vi "DAS_Hub.vi"() -> ()   [LabVIEW 2012]
uses:
  <vilib>/Platform/TimedLoop/XDataNode/timing_clust.ctl
  <vilib>/Platform/TimedLoop/XDataNode/nitl_modes.ctl
  <vilib>/Platform/TimedLoop/XDataNode/wakeup.ctl
  <vilib>/platform/TimedLoop/XDataNode/XDataNode.xnode
  <vilib>/regexp/Match Regular Expression.xnode
  <vilib>/Platform/TimedLoop/XDataNode/XDNodeRunTimeDep.lvlib
panel:
  in  "Pixel Size (uM)":dbl
  in  "Magnification":dbl
  in  "Time Between Shots":i64=200
  out "Most Recent Image":dbl[][](graph)
  in  "DAS MODE":u16(ring)=1 items=["Bulb Trigger Mode"=1, "Free Run Mode"=2]
  out "DER Host":bool
  out "DB Server":bool
  out "ProEM Host":bool
  out "ProEM Slave":bool
  out "CoolSnap Slave":bool
  out "PixelFly Slave":bool
  in  "Send To DER?":enum32{"Send to DER", "Don't Send to DER"}(radio)
  in  "Save as .AIA?":enum32{"Save to File", "Don't Save to File"}(radio)
  out "Top of Chamber Monitor":dynamicdata(graph)
  out "Atoms":i32[][](graph)
  in  "stop":bool
  out "Dark Field":i32[][](graph)
  out "No Atoms":i32[][](graph)
  # "(COMING SOON)"
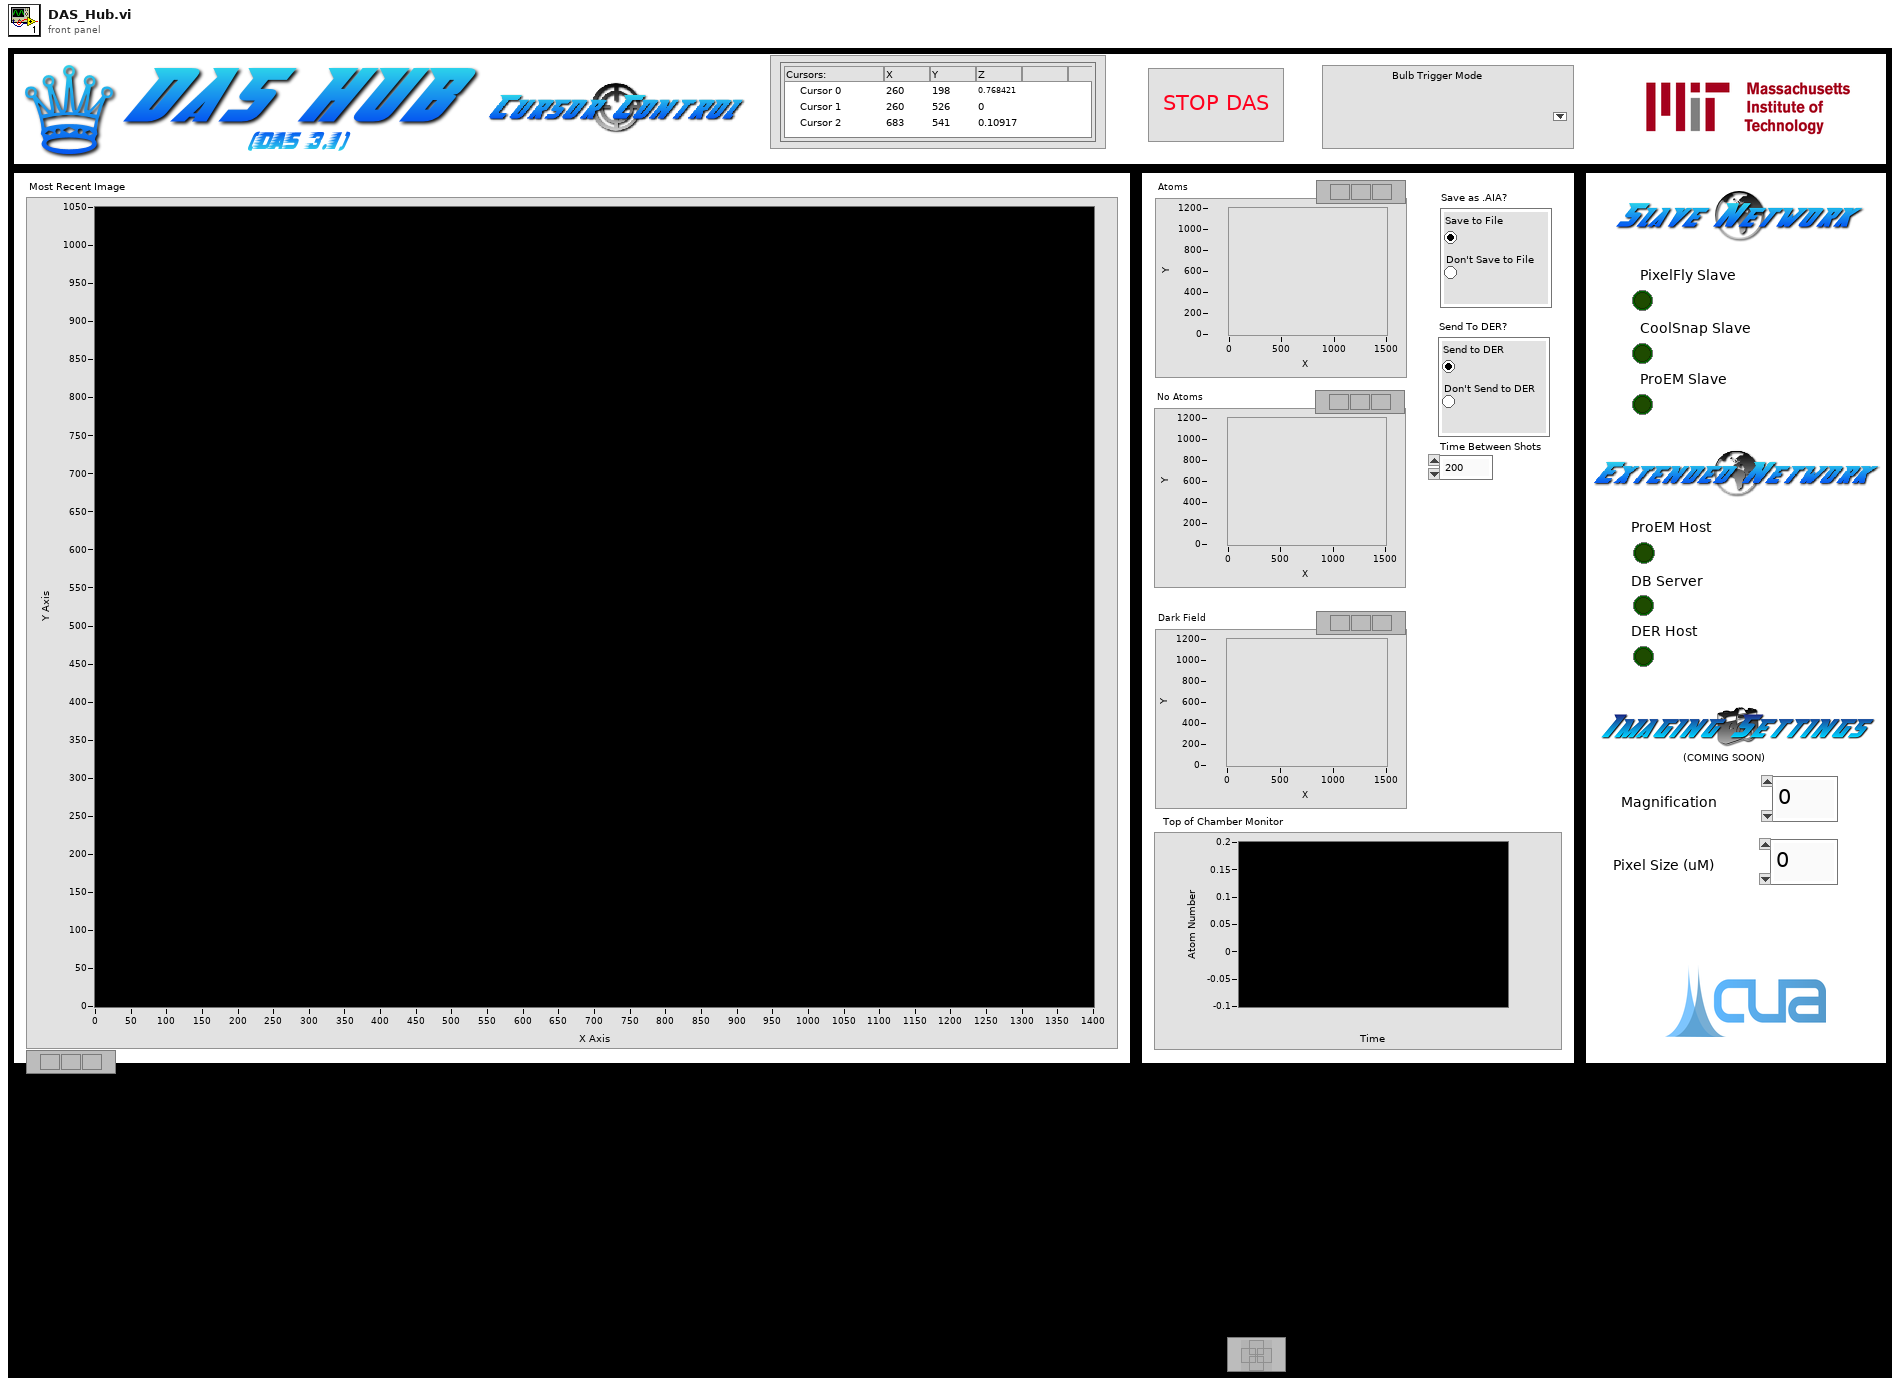
[diagram p1: front panel]
types:
  T1 = typedef "XDNodeRunTimeDep.lvlib/timing_clust.ctl" = cluster{"Expected End [f-1]":u64, "Actual End [f-1]":u64, "Finished Late? [f-1]":bool, "Expected End [i-1]":u64, "Actual End [i-1]":u64, "Finished Late? [i-1]":bool, "Expected Start [i]":u64, "Actual Start [i]":u64, "Expected Start [f]":u64, "Actual Start [f]":u64, "Source Name":string, "Structure Name":string, "Period":i64, "Deadline":i64, "Offset":i64, "Start":i64, "Priority":i32, "Timeout":i32, "Mode":T2, "Wakeup Reason":T3, "Error":errorcluster, "Source Type":string, "Secondary Source Type":string, "Global End Time":u64, "Global Start Time":u64, "Frame Duration":u64, "Iteration Duration":u64, "Assigned CPU":i32, "I/O Scan Engine Mode":u32}
  T2 = typedef "XDNodeRunTimeDep.lvlib/nitl_modes.ctl" = enum32{"No Change", "Process missed periods, maintain original phase", "Discard missed periods, maintain original phase", "Process missed periods, ignore original phase", "Discard missed periods, ignore original phase"}
  T3 = typedef "XDNodeRunTimeDep.lvlib/wakeup.ctl" = enum32{"Normal", "Aborted", "Asynchronous wakeup", "Timing source error", "Timed loop error", "Timeout"}
  T4 = typedef "LVDateTimeRec.ctl" = cluster{"fractional second":dbl, "second":i32, "minute":i32, "hour":i32, "day of month":i32, "month":i32, "year":i32, "day of week":i32, "day of year":i32, "DST":i32}
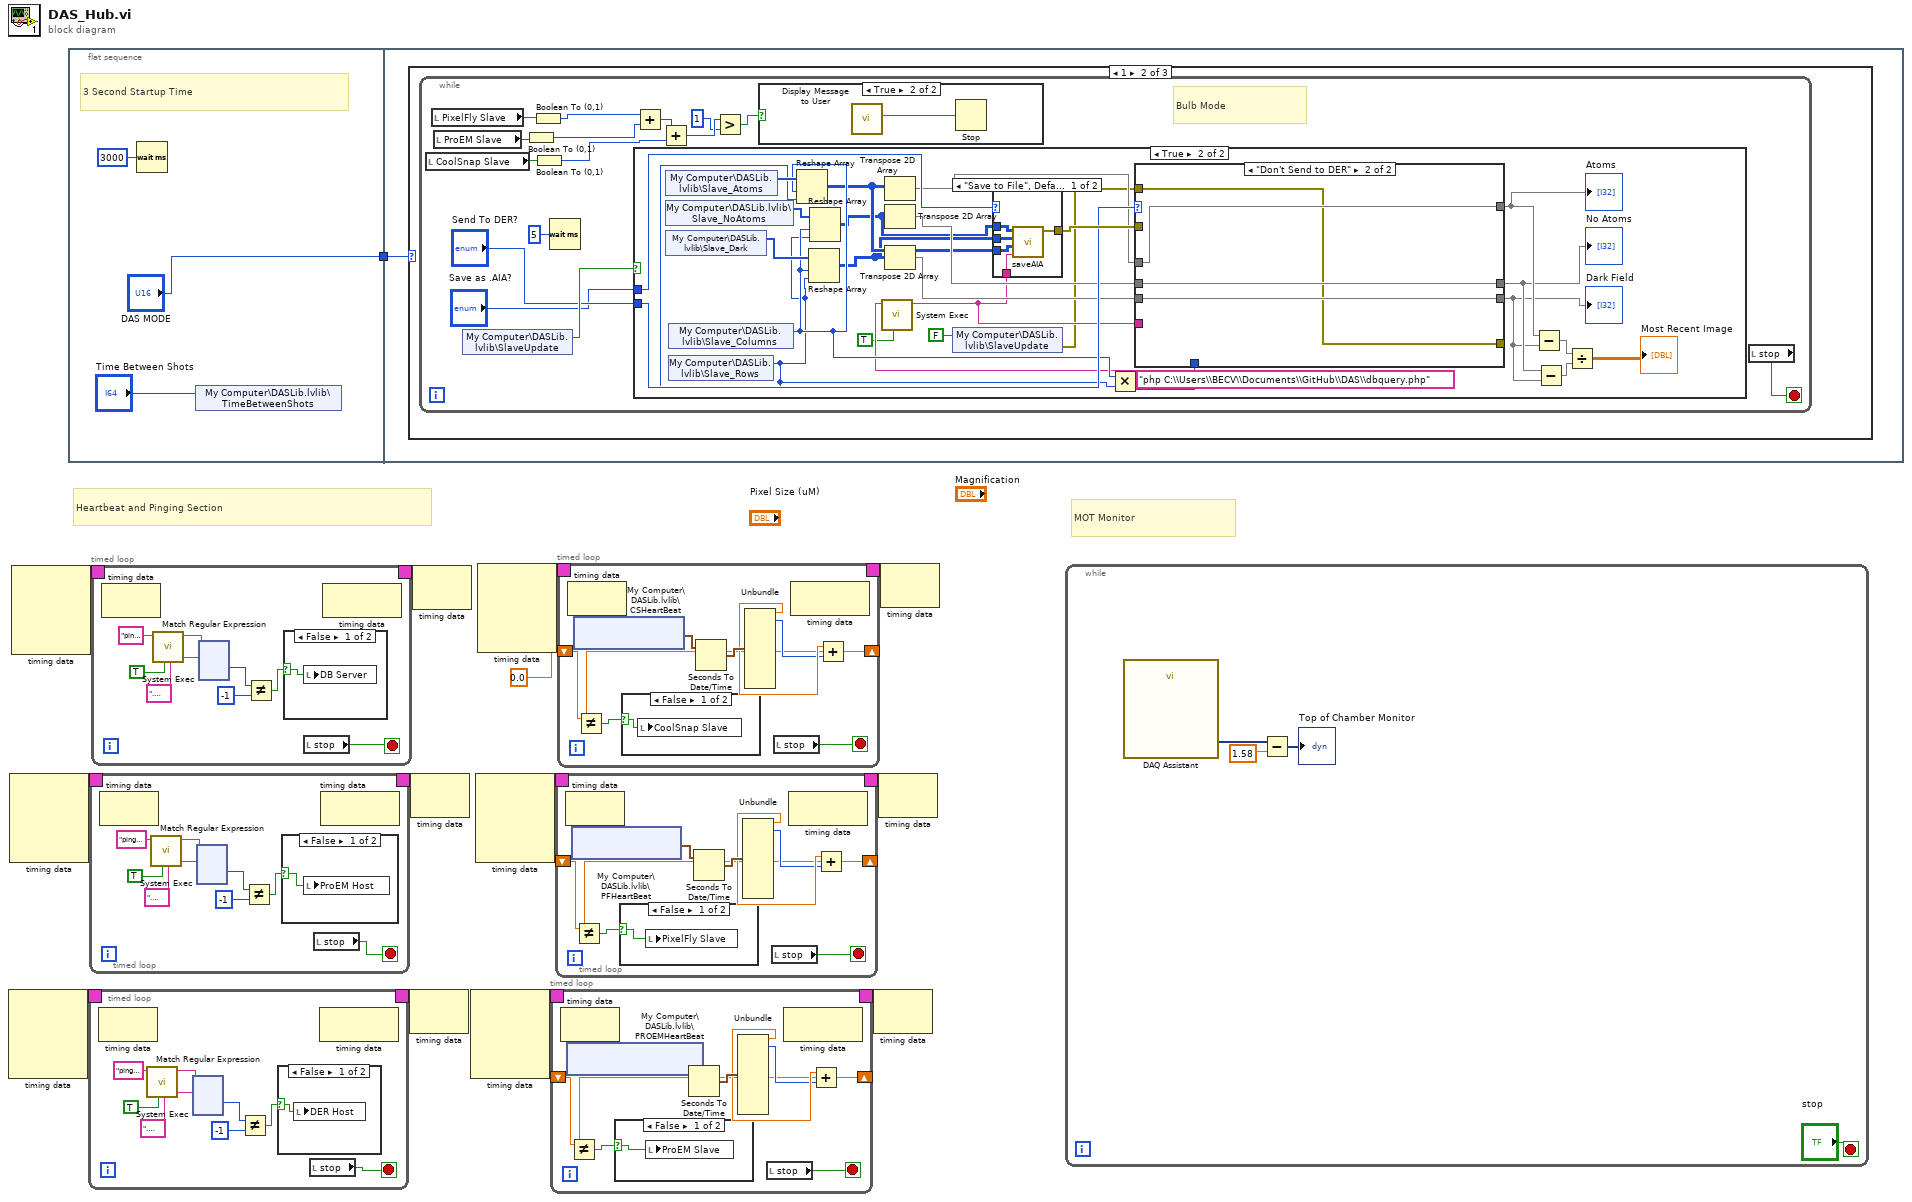
[diagram p0: block diagram]
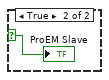
[diagram p2: hidden frame]
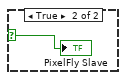
[diagram p3: hidden frame]
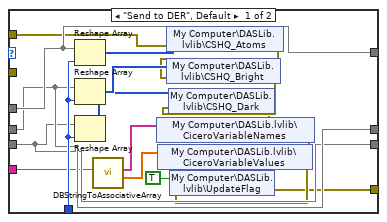
[diagram p7: hidden frame]
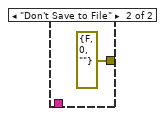
[diagram p8: hidden frame]
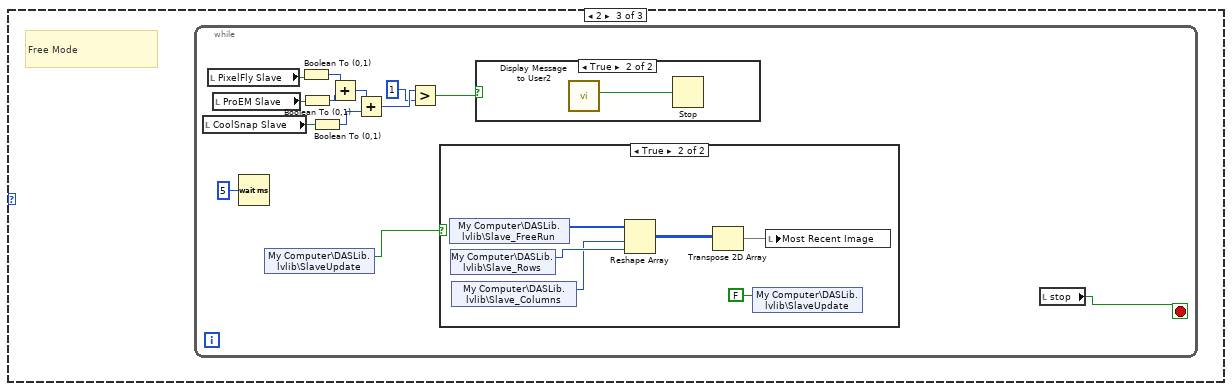
[diagram p9: hidden frame]
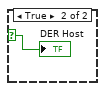
[diagram p12: hidden frame]
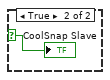
[diagram p13: hidden frame]
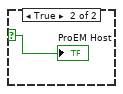
[diagram p14: hidden frame]
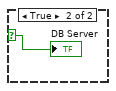
[diagram p15: hidden frame]
diagram:
  # "MOT Monitor"
  # "Heartbeat and Pinging Section"
  n1 = node-c288() -> (w8:T1)  [unwired: 4 in]
  n2 = node-c288() -> (w12:T1)  [unwired: 4 in]
  n3 = node-c288() -> (w14:T1)  [unwired: 4 in]
  n4 = flat-sequence {
    tunnel: ["DAS MODE"] -> w1
    tunnel: w1 -> [w18]
    frame #0 {
      # "3 Second Startup Time"
      n5 = Wait (ms)(milliseconds to wait=u32 3000) -> ()  [unwired: 1 out]
      n6 = shared-variable "My Computer\\DASLib.lvlib\\TimeBetweenShots"("Time Between Shots") -> ()  [unwired: 1 in, 1 out]
    }
    frame #1 {
      n7 = case shown="1" w18 {
        frame 0, Default {
          # "No-Camera Mode"
        }
        frame 1 {
          n8 = while {
            stop <- w29 stop-if-true
            # "Bulb Mode"
            n9 = local read "CoolSnap Slave"() -> (w26:bool)
            n10 = local read "PixelFly Slave"() -> (w28:bool)
            n11 = local read "ProEM Slave"() -> (w27:bool)
            n12 = shared-variable "My Computer\\DASLib.lvlib\\SlaveUpdate"() -> (w33:bool)  [unwired: 1 in, 1 out]
            n13 = Boolean To (0,1)(Boolean=w27) -> (0, 1=w24:i16)
            n14 = Boolean To (0,1)(Boolean=w28) -> (0, 1=w25:i16)
            n15 = Boolean To (0,1)(Boolean=w26) -> (0, 1=w23:i16)
            n16 = Wait (ms)(milliseconds to wait=u32 5) -> ()  [unwired: 1 out]
            n17 = case shown="True" w33 {
              tunnel: "Save as .AIA?" -> [_ w57]
              tunnel: "Send To DER?" -> [_ w55]
              frame False {
              }
              frame True {
                n18 = shared-variable "My Computer\\DASLib.lvlib\\Slave_Atoms"() -> (w60:i32[])  [unwired: 1 in, 1 out]
                n19 = shared-variable "My Computer\\DASLib.lvlib\\Slave_NoAtoms"() -> (w59:i32[])  [unwired: 1 in, 1 out]
                n20 = shared-variable "My Computer\\DASLib.lvlib\\Slave_Dark"() -> (w58:i32[])  [unwired: 1 in, 1 out]
                n21 = shared-variable "My Computer\\DASLib.lvlib\\Slave_Columns"() -> (w51:i32)  [unwired: 1 in, 1 out]
                n22 = shared-variable "My Computer\\DASLib.lvlib\\Slave_Rows"() -> (w50:i32)  [unwired: 1 in, 1 out]
                n23 = Reshape Array(w60, w51, w50) -> (w37:i32[][])
                n24 = Reshape Array(w58, w51, w50) -> (w36:i32[][])
                n25 = Reshape Array(w59, w51, w50) -> (w35:i32[][])
                n26 = call <vilib>:"System Exec.vi"("run minimized? (F)"=TRUE, "command line"="php C:\\Users\\BECV\\Documents\\GitHub\\DAS\\dbquery.php") -> ("standard output"=w41:string)  [unwired: 6 in, 3 out]
                n27 = Transpose 2D Array(2D array=w37) -> (transposed array=w54:i32[][])
                n28 = Transpose 2D Array(2D array=w35) -> (transposed array=w53:i32[][])
                n29 = Transpose 2D Array(2D array=w36) -> (transposed array=w52:i32[][])
                n30 = shared-variable "My Computer\\DASLib.lvlib\\SlaveUpdate"(FALSE ("SlaveUpdate")) -> (error out=w38:errorcluster)  [unwired: 1 in]
                n31 = case shown="\"Save to File\", Default" w57 {
                  tunnel: w35 -> [w87 _]
                  tunnel: w36 -> [w86 _]
                  tunnel: [w85 errorcluster {"status"=FALSE, "code"=0, "source"=""} ("error out")] -> w56
                  tunnel: w41 -> [w84 _]
                  tunnel: w37 -> [w83 _]
                  frame "Save to File", Default {
                    n32 = call "saveAIA.vi"("No Atoms"=w87, "Dark"=w86, "Atoms"=w83, "Db IN"=w84) -> ("error out"=w85:errorcluster)  [unwired: 6 in]
                  }
                  frame "Don't Save to File" {
                  }
                }
                n33 = Multiply(x=w51, y=w50) -> (x*y=w49:i32)
                n34 = case shown="\"Don't Send to DER\"" w55 {
                  tunnel: w56 -> [_ _]
                  tunnel: w54 -> [w71 w82]
                  tunnel: w53 -> [w70 w81]
                  tunnel: w52 -> [w69 w80]
                  tunnel: w49 -> [w78 _]
                  tunnel: [w71 w82] -> w48
                  tunnel: [w70 w81] -> w47
                  tunnel: [w69 w80] -> w46
                  tunnel: w41 -> [w68 _]
                  tunnel: [w62 w79] -> _
                  tunnel: w38 -> [w61 w79]
                  frame "Send to DER", Default {
                    n35 = Reshape Array(w71, w78) -> (w77:i32[])
                    n36 = Reshape Array(w70, w78) -> (w76:i32[])
                    n37 = Reshape Array(w69, w78) -> (w75:i32[])
                    n38 = call "DBStringToAssociativeArray.vi"("Raw DB String"=w68) -> ("Values"=w66:dbl[], "Names"=w67:string[])  [unwired: 9 in]
                    n39 = shared-variable "My Computer\\DASLib.lvlib\\CSHQ_Atoms"(w77, error in=w61) -> (error out=w74:errorcluster)
                    n40 = shared-variable "My Computer\\DASLib.lvlib\\CSHQ_Bright"(w76, error in=w74) -> (error out=w73:errorcluster)
                    n41 = shared-variable "My Computer\\DASLib.lvlib\\CSHQ_Dark"(w75, error in=w73) -> (error out=w65:errorcluster)
                    n42 = shared-variable "My Computer\\DASLib.lvlib\\CiceroVariableNames"(w67, error in=w65) -> (error out=w64:errorcluster)
                    n43 = shared-variable "My Computer\\DASLib.lvlib\\CiceroVariableValues"(w66, error in=w64) -> (error out=w63:errorcluster)
                    n44 = shared-variable "My Computer\\DASLib.lvlib\\UpdateFlag"(TRUE ("CSHQ_1_Changed"), error in=w63) -> (error out=w62:errorcluster)
                  }
                  frame "Don't Send to DER" {
                  }
                }
                "No Atoms" <- w47
                "Dark Field" <- w46
                "Atoms" <- w48
                n45 = Subtract(x=w48, y=w46) -> (x-y=w45:i32[][])
                n46 = Subtract(x=w47, y=w46) -> (x-y=w44:i32[][])
                n47 = Divide(x=w45, y=w44) -> (x/y=→"Most Recent Image":dbl[][])
              }
            }
            n48 = Add(x=w25, y=w24) -> (x+y=w22:i16)
            n49 = Add(x=w22, y=w23) -> (x+y=w21:i16)
            n50 = Greater?(x=w21, y=i16 1) -> (0:w19:bool)
            n51 = case shown="True" w19 {
              frame False {
              }
              frame True {
                n52 = call "Display Message to User"() -> ("OK"=w34:bool)  [unwired: 10 in, 1 out]
                n53 = Stop(stop? (T)=w34) -> ()
              }
            }
            n54 = local read "stop"() -> (w29:bool)
          }
        }
        frame 2 {
          # "Free Mode"
          n55 = while {
            stop <- w99 stop-if-true
            n56 = local read "CoolSnap Slave"() -> (w93:bool)
            n57 = local read "PixelFly Slave"() -> (w95:bool)
            n58 = local read "ProEM Slave"() -> (w94:bool)
            n59 = Wait (ms)(milliseconds to wait=u32 5) -> ()  [unwired: 1 out]
            n60 = shared-variable "My Computer\\DASLib.lvlib\\SlaveUpdate"() -> (w100:bool)  [unwired: 1 in, 1 out]
            n61 = Boolean To (0,1)(Boolean=w95) -> (0, 1=w90:i16)
            n62 = Boolean To (0,1)(Boolean=w94) -> (0, 1=w89:i16)
            n63 = Boolean To (0,1)(Boolean=w93) -> (0, 1=w92:i16)
            n64 = Add(x=w90, y=w89) -> (x+y=w91:i16)
            n65 = Add(x=w91, y=w92) -> (x+y=w98:i16)
            n66 = Greater?(x=w98, y=i16 1) -> (0:w96:bool)
            n67 = case shown="True" w100 {
              frame False {
              }
              frame True {
                n68 = shared-variable "My Computer\\DASLib.lvlib\\Slave_FreeRun"() -> (w107:i32[])  [unwired: 1 in, 1 out]
                n69 = shared-variable "My Computer\\DASLib.lvlib\\Slave_Rows"() -> (w106:i32)  [unwired: 1 in, 1 out]
                n70 = shared-variable "My Computer\\DASLib.lvlib\\Slave_Columns"() -> (w105:i32)  [unwired: 1 in, 1 out]
                n71 = Reshape Array(w107, w105, w106) -> (w104:i32[][])
                n72 = Transpose 2D Array(2D array=w104) -> (transposed array=w103:i32[][])
                n73 = shared-variable "My Computer\\DASLib.lvlib\\SlaveUpdate"(FALSE ("SlaveUpdate")) -> ()  [unwired: 1 in, 1 out]
                n74 = local write "Most Recent Image"(w103) -> ()
              }
            }
            n75 = case shown="True" w96 {
              frame False {
              }
              frame True {
                n76 = call "Display Message to User2"() -> ("OK"=w102:bool)  [unwired: 10 in, 1 out]
                n77 = Stop(stop? (T)=w102) -> ()
              }
            }
            n78 = local read "stop"() -> (w99:bool)
          }
        }
      }
    }
  }
  n79 = timed-loop {
    timing: w8 -> [_]
    timing-out: [_] -> w7
    stop <- w116 stop-if-true
    n80 = node-c288() -> ()  [unwired: 1 in, 1 out]
    n81 = call <vilib>:"System Exec.vi"("run minimized? (F)"=TRUE, "command line"="ping 192.168.1.185 -n 1") -> ("standard output"=w113:string)  [unwired: 6 in, 3 out]
    n82 = xnode "Match Regular Expression"("input string"=w113, "regular expression"=".*[0-9]+ms") -> ("offset past match"=w111:i32)  [unwired: 4 in, 4 out]
    n83 = Not Equal?(x=w111, y=-1) -> (x != y?=w109:bool)
    n84 = case shown="False" w109 {
      selector: w109 -> [w117 w118]
      frame False {
        n85 = local write "DER Host"(w117) -> ()
      }
      frame True {
        "DER Host" <- w118
      }
    }
    n86 = local read "stop"() -> (w116:bool)
    n87 = node-c288() -> ()  [unwired: 1 in, 1 out]
  }
  n88 = timed-loop {
    timing: w12 -> [_]
    timing-out: [_] -> w11
    stop <- w239 stop-if-true
    n89 = node-c288() -> ()  [unwired: 1 in, 1 out]
    n90 = call <vilib>:"System Exec.vi"("run minimized? (F)"=TRUE, "command line"="ping 192.168.1.135 -n 1") -> ("standard output"=w236:string)  [unwired: 6 in, 3 out]
    n91 = xnode "Match Regular Expression"("input string"=w236, "regular expression"=".*[0-9]+ms") -> ("offset past match"=w234:i32)  [unwired: 4 in, 4 out]
    n92 = Not Equal?(x=w234, y=-1) -> (x != y?=w232:bool)
    n93 = case shown="False" w232 {
      selector: w232 -> [w240 w241]
      frame False {
        n94 = local write "ProEM Host"(w240) -> ()
      }
      frame True {
        "ProEM Host" <- w241
      }
    }
    n95 = local read "stop"() -> (w239:bool)
    n96 = node-c288() -> ()  [unwired: 1 in, 1 out]
  }
  n97 = timed-loop {
    timing: w14 -> [_]
    timing-out: [_] -> w13
    stop <- w362 stop-if-true
    n98 = node-c288() -> ()  [unwired: 1 in, 1 out]
    n99 = call <vilib>:"System Exec.vi"("run minimized? (F)"=TRUE, "command line"="ping 192.168.1.227 -n 1") -> ("standard output"=w359:string)  [unwired: 6 in, 3 out]
    n100 = xnode "Match Regular Expression"("input string"=w359, "regular expression"=".*[0-9]+ms") -> ("offset past match"=w357:i32)  [unwired: 4 in, 4 out]
    n101 = Not Equal?(x=w357, y=-1) -> (x != y?=w355:bool)
    n102 = case shown="False" w355 {
      selector: w355 -> [w363 w364]
      frame False {
        n103 = local write "DB Server"(w363) -> ()
      }
      frame True {
        "DB Server" <- w364
      }
    }
    n104 = local read "stop"() -> (w362:bool)
    n105 = node-c288() -> ()  [unwired: 1 in, 1 out]
  }
  n106 = node-c288(w7) -> ()  [unwired: 1 out]
  n107 = node-c288(w11) -> ()  [unwired: 1 out]
  n108 = node-c288(w13) -> ()  [unwired: 1 out]
  n109 = node-c288() -> (w3:T1)  [unwired: 4 in]
  n110 = node-c288() -> (w5:T1)  [unwired: 4 in]
  n111 = node-c288() -> (w10:T1)  [unwired: 4 in]
  n112 = timed-loop {
    timing: w3 -> [_]
    timing-out: [_] -> w2
    shift-right: [w479] -> _
    shift-left: _ -> [w480]
    stop <- w485 stop-if-true
    n113 = node-c288() -> ()  [unwired: 1 in, 1 out]
    n114 = shared-variable "My Computer\\DASLib.lvlib\\PROEMHeartBeat"() -> (w484:timestamp)  [unwired: 1 in, 2 out]
    n115 = Seconds To Date/Time(time stamp (now)=w484) -> (date time rec=w483:T4)  [unwired: 1 in]
    n116 = Unbundle(w483) -> ("fractional second"=w482:dbl, "second"=w481:i32)  [unwired: 8 out]
    n117 = local read "stop"() -> (w485:bool)
    n118 = node-c288() -> ()  [unwired: 1 in, 1 out]
    n119 = Add(x=w482, y=w481) -> (x+y=w479:dbl)
    n120 = Not Equal?(x=w480, y=w479) -> (x != y?=w478:bool)
    n121 = case shown="False" w478 {
      selector: w478 -> [w486 w487]
      frame False {
        n122 = local write "ProEM Slave"(w486) -> ()
      }
      frame True {
        "ProEM Slave" <- w487
      }
    }
  }
  n123 = timed-loop {
    timing: w5 -> [_]
    timing-out: [_] -> w4
    shift-right: [w491] -> _
    shift-left: _ -> [w492]
    stop <- w497 stop-if-true
    n124 = node-c288() -> ()  [unwired: 1 in, 1 out]
    n125 = shared-variable "My Computer\\DASLib.lvlib\\PFHeartBeat"() -> (w496:timestamp)  [unwired: 1 in, 2 out]
    n126 = Seconds To Date/Time(time stamp (now)=w496) -> (date time rec=w495:T4)  [unwired: 1 in]
    n127 = Unbundle(w495) -> ("fractional second"=w494:dbl, "second"=w493:i32)  [unwired: 8 out]
    n128 = local read "stop"() -> (w497:bool)
    n129 = node-c288() -> ()  [unwired: 1 in, 1 out]
    n130 = Add(x=w494, y=w493) -> (x+y=w491:dbl)
    n131 = Not Equal?(x=w492, y=w491) -> (x != y?=w490:bool)
    n132 = case shown="False" w490 {
      selector: w490 -> [w498 w499]
      frame False {
        n133 = local write "PixelFly Slave"(w498) -> ()
      }
      frame True {
        "PixelFly Slave" <- w499
      }
    }
  }
  n134 = timed-loop {
    timing: w10 -> [_]
    timing-out: [_] -> w9
    shift-right: [w503] -> _
    shift-left: 0.0 -> [w504]
    stop <- w509 stop-if-true
    n135 = node-c288() -> ()  [unwired: 1 in, 1 out]
    n136 = shared-variable "My Computer\\DASLib.lvlib\\CSHeartBeat"() -> (w508:timestamp)  [unwired: 1 in, 2 out]
    n137 = Seconds To Date/Time(time stamp (now)=w508) -> (date time rec=w507:T4)  [unwired: 1 in]
    n138 = Unbundle(w507) -> ("fractional second"=w506:dbl, "second"=w505:i32)  [unwired: 8 out]
    n139 = local read "stop"() -> (w509:bool)
    n140 = node-c288() -> ()  [unwired: 1 in, 1 out]
    n141 = Add(x=w506, y=w505) -> (x+y=w503:dbl)
    n142 = Not Equal?(x=w504, y=w503) -> (x != y?=w502:bool)
    n143 = case shown="False" w502 {
      selector: w502 -> [w510 w511]
      frame False {
        n144 = local write "CoolSnap Slave"(w510) -> ()
      }
      frame True {
        "CoolSnap Slave" <- w511
      }
    }
  }
  n145 = node-c288(w2) -> ()  [unwired: 1 out]
  n146 = node-c288(w4) -> ()  [unwired: 1 out]
  n147 = node-c288(w9) -> ()  [unwired: 1 out]
  n148 = while {
    stop <- "stop" stop-if-true
    n149 = call "DAQ Assistant"() -> ("data"=w516:dynamicdata)  [unwired: 17 in, 2 out]
    n150 = Subtract(x=w516, y=1.58) -> (x-y=→"Top of Chamber Monitor":dynamicdata)
  }
